vi "Write Data.vi"(8 "error in (no error)":errorcluster, 9 "Publication Time":timestamp, 10 "Value":variant, 11 "QueueTransport In":refnum<class "QueueTransport.lvclass">) -> (0 "error out":errorcluster, 3 "QueueTransport Out":refnum<class "QueueTransport.lvclass">)   [LabVIEW 2015, in "Mediator.lvlib" / "QueueTransport.lvclass"]
doc: "<License>\nCopyright © 2017 Composed Systems, LLC | All rights reserved\nwww.composed.io\n\nAuthor: Ethan Stern <ethan.stern@composed.io>\n\nThis software is provided \"AS IS\" WITHOUT WARRANTIES, either express or implied, AND IS FOR EDUCATIONAL PURPOSES ONLY.\n</License>"
uses:
  QueueTransport.lvclass
  QueueTransport.lvclass/QueueTransport.ctl
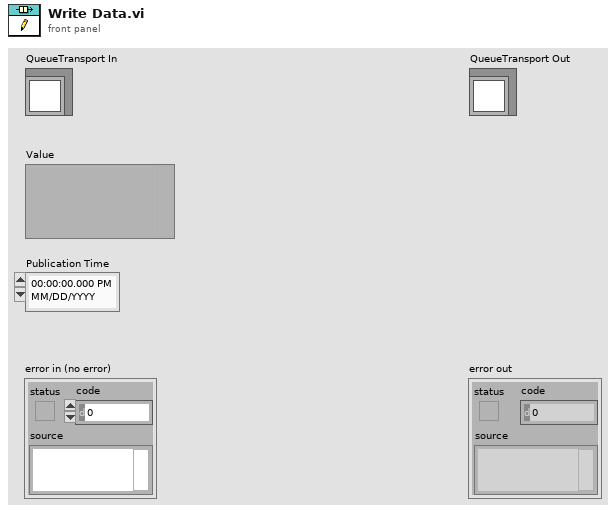
[diagram p1: front panel]
types:
  T1 = cluster{"Value":variant, "Publication Time":timestamp}
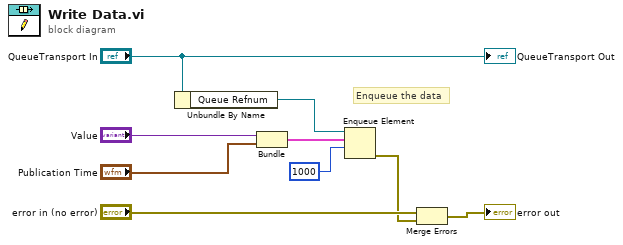
[diagram p0: block diagram]
diagram:
  # "Enqueue the data"
  n1 = Unbundle By Name("QueueTransport In") -> ("Queue Refnum"=w8:refnum<queue>)
  n2 = Bundle("Value"="Value", "Publication Time"="Publication Time") -> (w2:T1)  [unwired: 1 in]
  n3 = Enqueue Element(queue=w8, element=w2, timeout in ms (-1)=1000) -> (error out=w5:errorcluster)  [unwired: 1 in, 2 out]
  n4 = Merge Errors("error in (no error)", w5) -> (→"error out":errorcluster)
  "QueueTransport Out" <- "QueueTransport In"
